vi "CreateBufferAndAdd.vi"(8 "error in (no error)":errorcluster, 9 "Size in Bytes":u64, 10 "Buffer Name":string, 11 "Buffers":T1[](array[typedef])) -> (0 "error out":errorcluster, 2 "output buffer":T1, 3 "output buffers":T1[](array[typedef]))   [LabVIEW 2016]
uses:
  private/vis/BufferStruct.ctl
panel:
  in  "buffer":T1
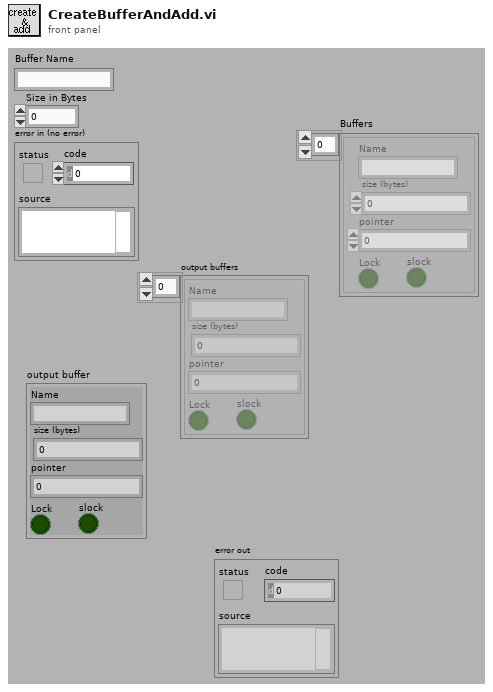
[diagram p1: front panel]
types:
  T1 = typedef "BufferStruct.ctl" = cluster{"Name":string, "size (bytes)":u64, "pointer":u64, "Lock":bool, "slock":bool}
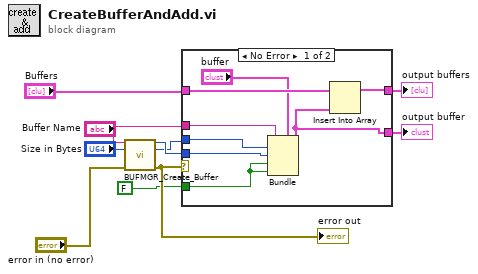
[diagram p0: block diagram]
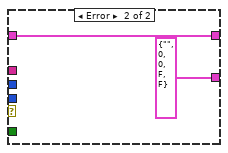
[diagram p2: hidden frame]
diagram:
  n1 = call "BUFMGR_Create_Buffer.vi"("Buffer Name"="Buffer Name", "Size in Bytes"="Size in Bytes", "error in (no error)"="error in (no error)") -> ("pointer to buff"=w3:u64, "Size in Bytes out"=w2:u64, "error out"=w8:errorcluster)  [unwired: 10 out]
  "error out" <- w8
  n2 = case shown="No Error" w8 {
    tunnel: "Buffer Name" -> [w18 _]
    tunnel: w2 -> [w17 _]
    tunnel: w3 -> [w16 _]
    tunnel: FALSE -> [w12 _]
    tunnel: [w14 w20] -> w6
    tunnel: "Buffers" -> [w15 w20]
    tunnel: [w11 T1 {"Name"="", "size (bytes)"=0, "pointer"=0, "Lock"=FALSE, "slock"=FALSE} ("output buffer")] -> w1
    frame No Error {
      n3 = Bundle(cluster="buffer", "Name"=w18, "size (bytes)"=w17, "pointer"=w16, "Lock"=w12, "slock"=w12) -> (w11:T1)
      n4 = Insert Into Array(array=w15, new element=w11) -> (w14:T1[])  [unwired: 1 in]
    }
    frame Error {
    }
  }
  "output buffers" <- w6
  "output buffer" <- w1
